vi "TopLevel.vi"() -> ()   [LabVIEW 2021]
uses:
  <vilib>/Platform/TimedLoop/XDataNode/wakeup.ctl
  <vilib>/Platform/TimedLoop/XDataNode/XDNodeRunTimeDep.lvlib
  <vilib>/Platform/TimedLoop/XDataNode/nitl_modes.ctl
  <vilib>/Platform/TimedLoop/XDataNode/timing_clust.ctl
  <vilib>/platform/TimedLoop/XDataNode/XDataNode.xnode
  <vilib>/rvi/FXPMathLib/basic elements/FxpDiscreteDelay/XNode/nifxpmath_DiscreteDelay.xnode
panel:
  out "IO.ReferenceDesignOUT5":u8
  out "IO.ReferenceDesignOUT4":u8
  in  "IO.ReferenceDesignIN5":u8
  in  "IO.ReferenceDesignIN4":u8
  out "IO.ReferenceDesignOUT3":u8
  out "IO.ReferenceDesignOUT2":u8
  out "IO.ReferenceDesignOUT1":u8
  in  "IO.ReferenceDesignIN3":u8
  in  "IO.ReferenceDesignIN2":u8
  in  "IO.ReferenceDesignIN1":u8
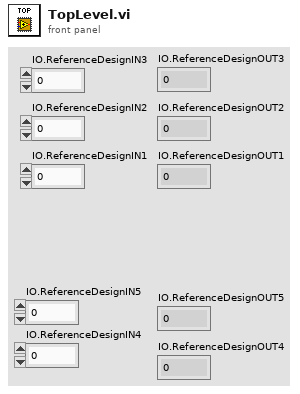
[diagram p1: front panel]
types:
  T1 = typedef "XDNodeRunTimeDep.lvlib/timing_clust.ctl" = cluster{"Expected End [f-1]":u64, "Actual End [f-1]":u64, "Finished Late? [f-1]":bool, "Expected End [i-1]":u64, "Actual End [i-1]":u64, "Finished Late? [i-1]":bool, "Expected Start [i]":u64, "Actual Start [i]":u64, "Expected Start [f]":u64, "Actual Start [f]":u64, "Source Name":string, "Structure Name":string, "Period":i64, "Deadline":i64, "Offset":i64, "Start":i64, "Priority":i32, "Timeout":i32, "Mode":T2, "Wakeup Reason":T3, "Error":errorcluster, "Source Type":string, "Secondary Source Type":string, "Global End Time":u64, "Global Start Time":u64, "Frame Duration":u64, "Iteration Duration":u64, "Assigned CPU":i32, "I/O Scan Engine Mode":u32}
  T2 = typedef "XDNodeRunTimeDep.lvlib/nitl_modes.ctl" = enum32{"No Change", "Process missed periods, maintain original phase", "Discard missed periods, maintain original phase", "Process missed periods, ignore original phase", "Discard missed periods, ignore original phase"}
  T3 = typedef "XDNodeRunTimeDep.lvlib/wakeup.ctl" = enum32{"Normal", "Aborted", "Asynchronous wakeup", "Timing source error", "Timed loop error", "Timeout"}
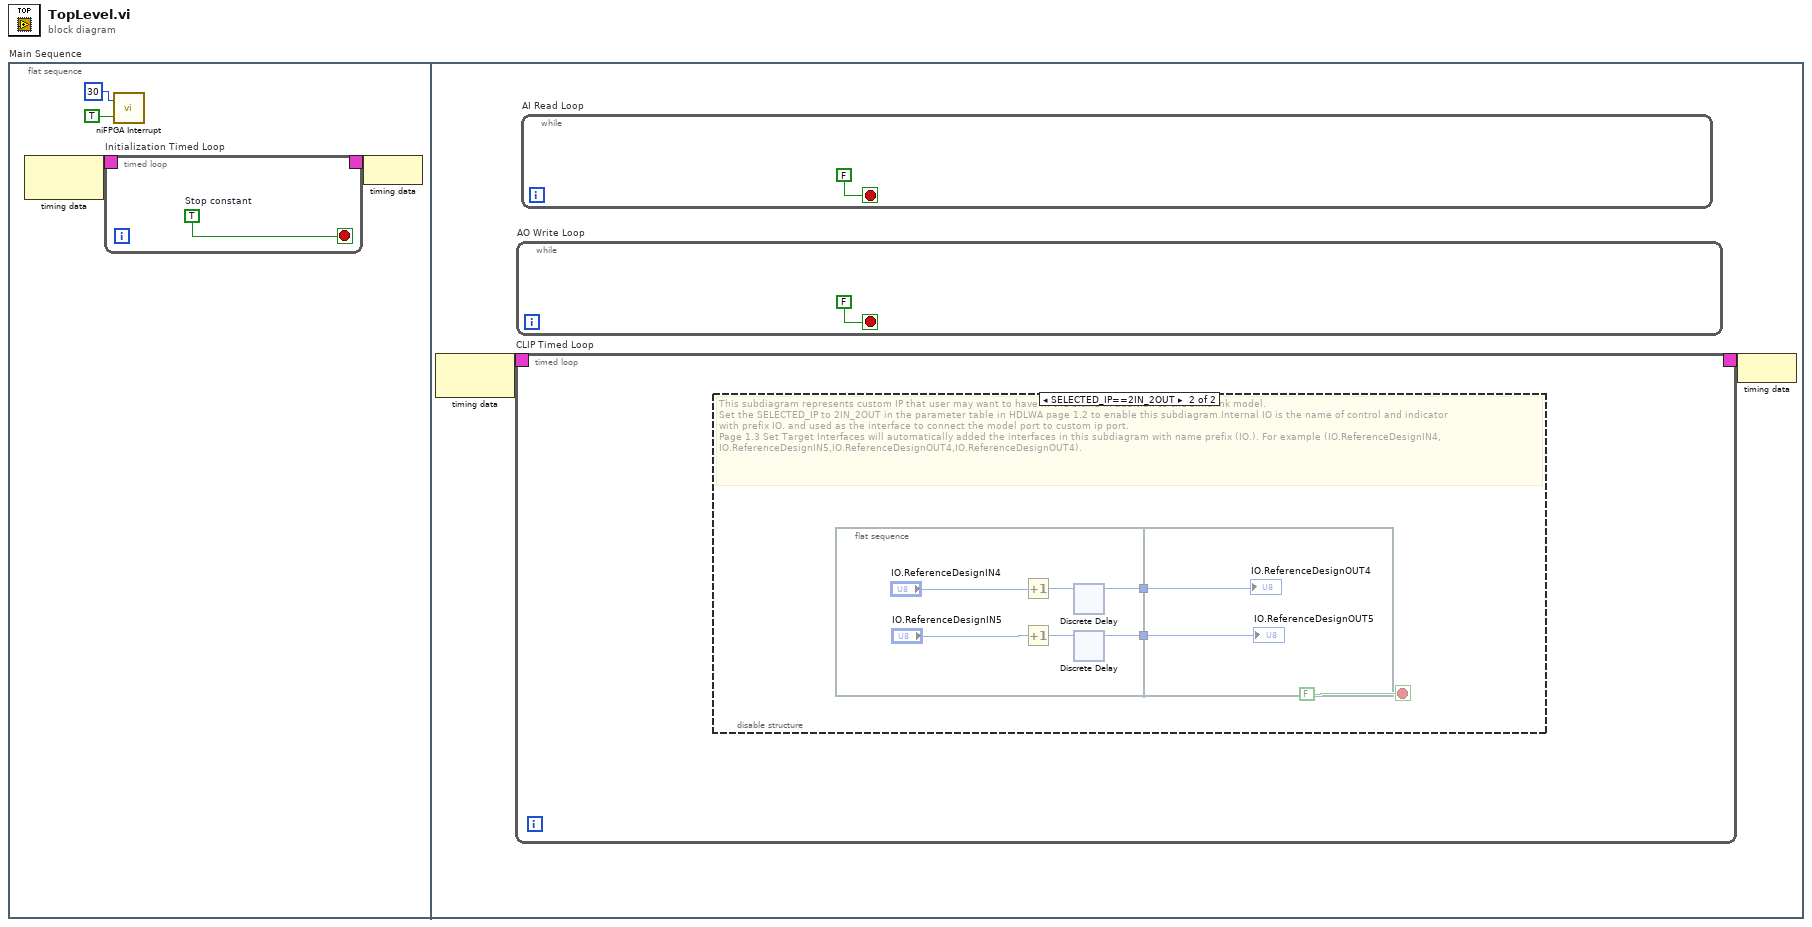
[diagram p0: block diagram]
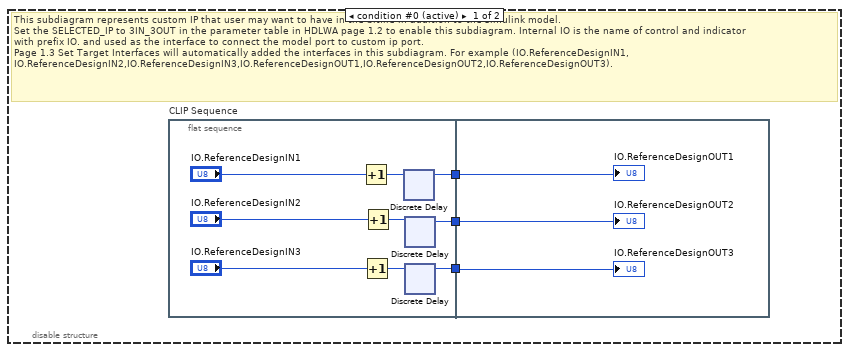
[diagram p2: hidden frame]
diagram:
  n1 = flat-sequence "Main Sequence" {
    frame #0 {
      n2 = node-c288 ("Input Node")() -> (w2:T1)  [unwired: 1 in]
      n3 = timed-loop "Initialization Timed Loop" {
        timing: w2 -> [_]
        timing-out: [_] -> w1
        stop <- w5 stop-if-true
        w5 = TRUE  # Stop constant
      }
      n4 = call <vilib>:"niFPGA Interrupt.vi"("Wait Until Cleared (F)"=TRUE, "IRQ Number (0)"=u8 30) -> ()  [unwired: 1 in]
      n5 = node-c288 ("Output Node")(w1) -> ()
    }
    frame #1 {
      n6 = node-c288 ("Input Node")() -> (w11:T1)  [unwired: 1 in]
      n7 = timed-loop "CLIP Timed Loop" {
        timing: w11 -> [_]
        timing-out: [_] -> w10
        stop <- FALSE stop-if-true
        n8 = disable-structure shown="SELECTED_IP==2IN_2OUT" {
          frame condition #0 (active) {
            # "This subdiagram represents custom IP that user may want to have in the bitfile in addition to the simulink model.\nSet the SELECTED_IP to 3IN_3OUT in the parameter table in HDLWA page 1.2 to enable this subdiagram. Internal IO is the name of control and indicator\nwith prefix IO. and used as the interface to connect the model port to custom ip port.\nPage 1.3 Set Target Interfaces will automatically added the interfaces in this subdiagram. For example (IO.ReferenceDesignIN1,\nIO.ReferenceDesignIN2,IO.ReferenceDesignIN3,IO.ReferenceDesignOUT1,IO.ReferenceDesignOUT2,IO.ReferenceDesignOUT3)."
            n9 = flat-sequence "CLIP Sequence" {
              tunnel: [w19] -> w16
              tunnel: [w18] -> w15
              tunnel: [w17] -> w14
              tunnel: w16 -> [w28]
              tunnel: w15 -> [w27]
              tunnel: w14 -> [w26]
              frame #0 {
                n10 = Increment(x="IO.ReferenceDesignIN1") -> (x+1=w25:u8)
                n11 = Increment(x="IO.ReferenceDesignIN3") -> (x+1=w21:u8)
                n12 = Increment(x="IO.ReferenceDesignIN2") -> (x+1=w22:u8)
                n13 = xnode ("Discrete Delay")("D"=w25) -> ("Q"=w17:u8)
                n14 = xnode ("Discrete Delay")("D"=w22) -> ("Q"=w18:u8)
                n15 = xnode ("Discrete Delay")("D"=w21) -> ("Q"=w19:u8)
              }
              frame #1 {
                "IO.ReferenceDesignOUT3" <- w28
                "IO.ReferenceDesignOUT2" <- w27
                "IO.ReferenceDesignOUT1" <- w26
              }
            }
          }
          frame condition #1 {
            # "This subdiagram represents custom IP that user may want to have in the bitfile in addition to the simulink model.\nSet the SELECTED_IP to 2IN_2OUT in the parameter table in HDLWA page 1.2 to enable this subdiagram.Internal IO is the name of control and indicator\nwith prefix IO. and used as the interface to connect the model port to custom ip port.\nPage 1.3 Set Target Interfaces will automatically added the interfaces in this subdiagram with name prefix (IO.). For example (IO.ReferenceDesignIN4,\nIO.ReferenceDesignIN5,IO.ReferenceDesignOUT4,IO.ReferenceDesignOUT4)."
            n16 = flat-sequence {
              tunnel: [w32] -> w30
              tunnel: [w31] -> w29
              tunnel: w30 -> [w38]
              tunnel: w29 -> [w37]
              frame #0 {
                n17 = Increment(x="IO.ReferenceDesignIN4") -> (x+1=w35:u8)
                n18 = Increment(x="IO.ReferenceDesignIN5") -> (x+1=w34:u8)
                n19 = xnode ("Discrete Delay")("D"=w35) -> ("Q"=w31:u8)
                n20 = xnode ("Discrete Delay")("D"=w34) -> ("Q"=w32:u8)
              }
              frame #1 {
                "IO.ReferenceDesignOUT5" <- w38
                "IO.ReferenceDesignOUT4" <- w37
              }
            }
          }
        }
      }
      n21 = while "AO Write Loop" {
        stop <- FALSE stop-if-true
      }
      n22 = while "AI Read Loop" {
        stop <- FALSE stop-if-true
      }
      n23 = node-c288 ("Output Node")(w10) -> ()
    }
  }
